vi "BioFeedback7(DAQ+8-channel)SubVIToUI.vi"(0 "UI Data Input File":path=path "C:/Users/Tinggroup/Desktop/VRMuscleActivationVisualizer/StationaryVisualFeedbackVR/assets/BiofeedbackData.txt", 7 "Frames Per Second":dbl=30.0, 9 "Start Trial":bool, 11 "End Trial":bool, 12 "Data Directory":path, 13 "File Name":string, 14 "Extension":string="_EMG.txt") -> ()   [LabVIEW 2016]
uses:
  <vilib>/Utility/error.llb/DialogType.ctl
  <vilib>/Analysis/5stat.llb/RMS (DBL).vi
  <vilib>/Waveform/WDTFileIO.llb/Export Waveform To Spreadsheet File.vi
  <vilib>/Waveform/WDTOps.llb/WDT Append Waveforms DBL.vi
  <vilib>/Analysis/NI_AALPro.lvlib
  <resource>/objmgr/daqmx.rc
panel:
  in  "EMG Input Device\nProduct Type":string
  out "Moving Avg 1AND2":dbl(slide) scale=0.0..0.01
  out "Moving Avg 3AND4":dbl(slide) scale=0.5..0.7
  out "RMS 3AND4":dbl(graph)
  out "RMS 1AND2":dbl(graph)
  out "RMS 8":dbl(graph)
  out "RMS 7":dbl(graph)
  out "RMS 6":dbl(graph)
  out "RMS 5":dbl(graph)
  out "RMS 4":dbl(graph)
  out "RMS 3":dbl(graph)
  out "RMS 2":dbl(graph)
  out "RMS 1":dbl(graph)
  out "Aggregate8":waveform(dbl)[](array[waveform])
  out "Aggregate7":waveform(dbl)[](array[waveform])
  out "Aggregate6":waveform(dbl)[](array[waveform])
  out "Aggregate5":waveform(dbl)[](array[waveform])
  out "Aggregate4":waveform(dbl)[](array[waveform])
  out "Aggregate3":waveform(dbl)[](array[waveform])
  out "Aggregate2":waveform(dbl)[](array[waveform])
  out "Aggregate1":waveform(dbl)[](array[waveform])
  out "Wfm8":waveform(dbl)
  out "Wfm7":waveform(dbl)
  out "Wfm6":waveform(dbl)
  out "Wfm5":waveform(dbl)
  out "Wfm4":waveform(dbl)
  out "Wfm3":waveform(dbl)
  out "Wfm2":waveform(dbl)
  out "Wfm1":waveform(dbl)
  out "Trial Data":waveform(dbl)(graph)
  in  "UI Percent Path":path=path "C:/Users/Tinggroup/Desktop/VRMuscleActivationVisualizer/StationaryVisualFeedbackVR/assets/BiofeedbackTargetPercentage.txt"
  in  "Target Percentage":dbl
  out "Trial In Progress":bool
  in  "Trial Number":dbl
  in  "MARK":bool
  out "Moving Avg RMS Graph":dbl(graph)
  out "Moving Avg RMS":dbl(slide) scale=0.0..2.0
  in  "Lower Cut-Off":dbl=20.0
  in  "Upper Cut-Off":dbl=300.0
  out "raw data":dynamicdata(graph)
  out "Bufffer Index":dbl
  out "Frames in Buffer":dbl
  out "Samples per frame":dbl
  out "Reset Data Acquisition\nAnd UI Updating":bool=TRUE
  in  "Moving Average Length (s)":dbl=0.5
  in  "Sample rate (Hz)":dbl=2000.0
  in  "End Program":bool
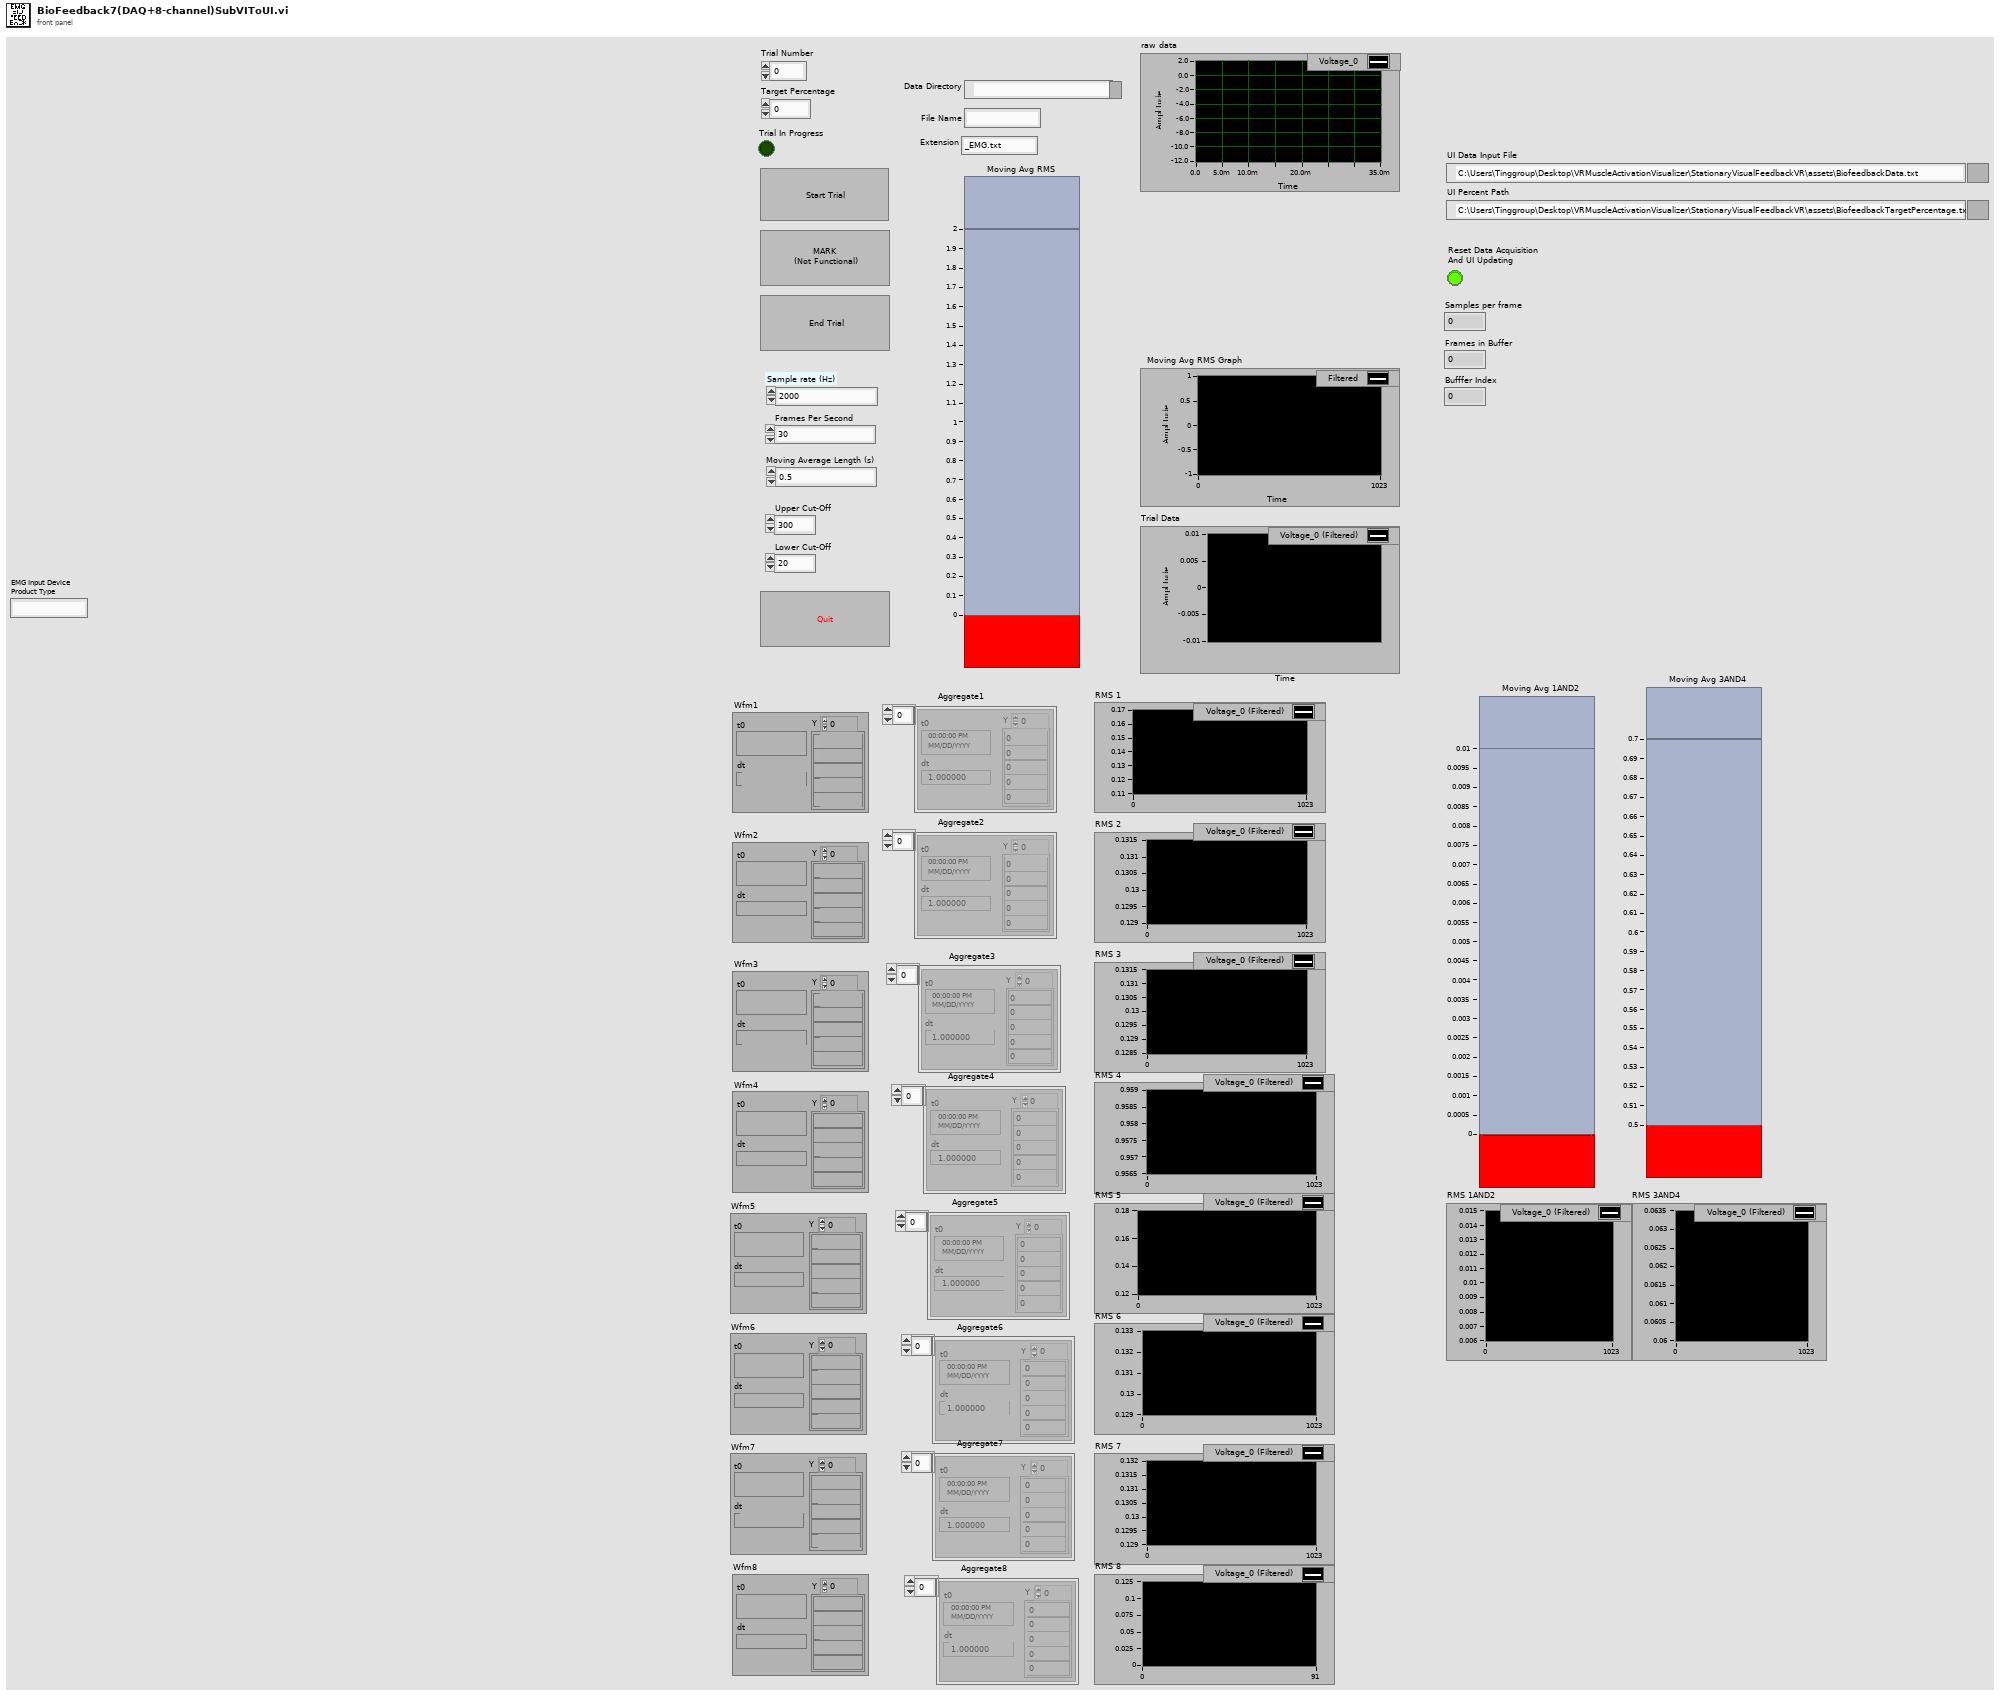
[diagram p1: front panel]
types:
  T1 = typedef "DialogType.ctl" = u16
  T2 = typedef "WaveformArrayControl.ctl" = waveform(dbl)[]
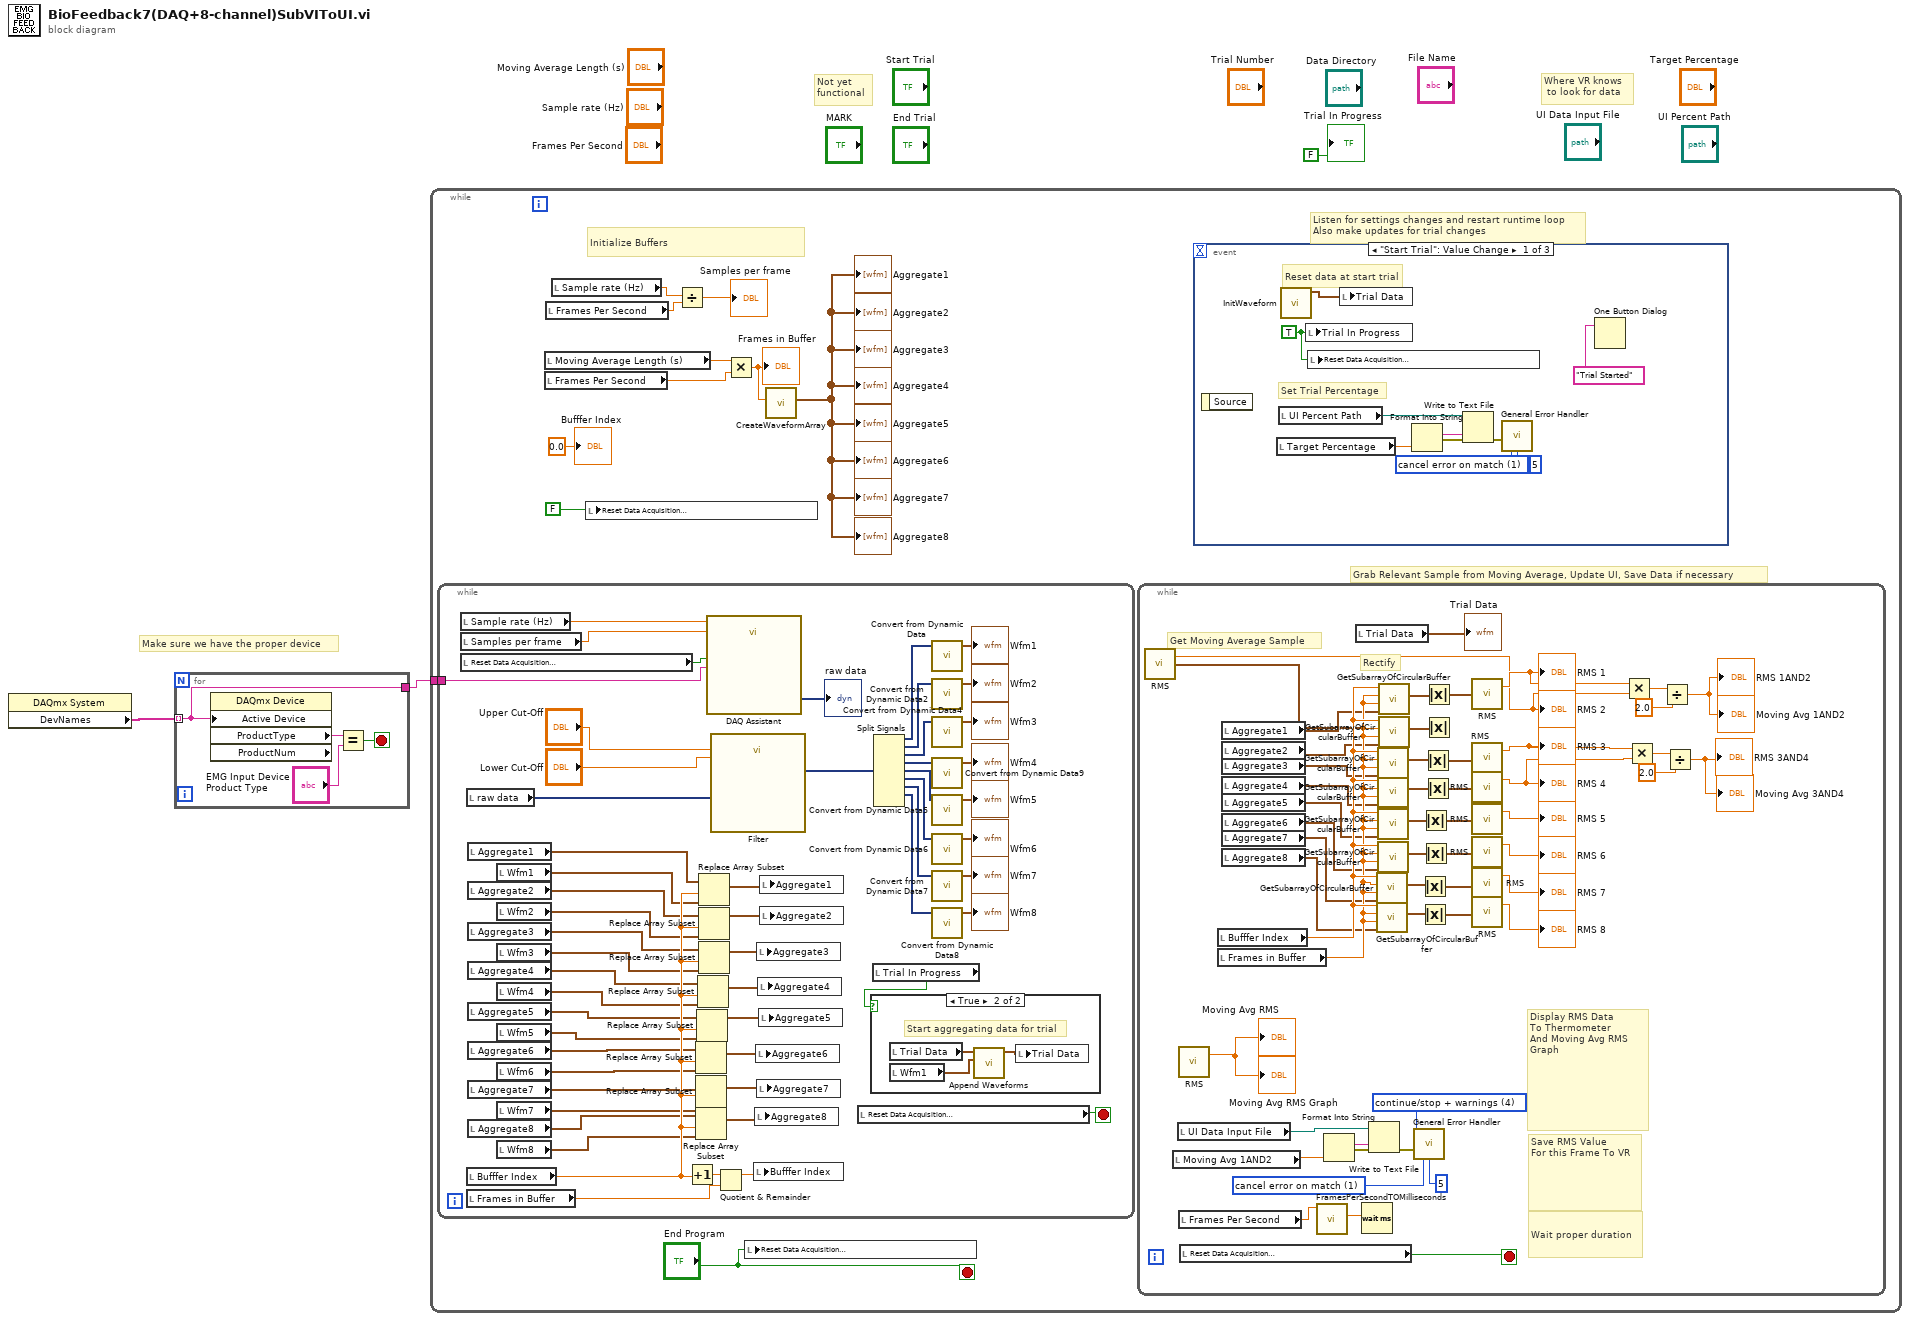
[diagram p0: block diagram]
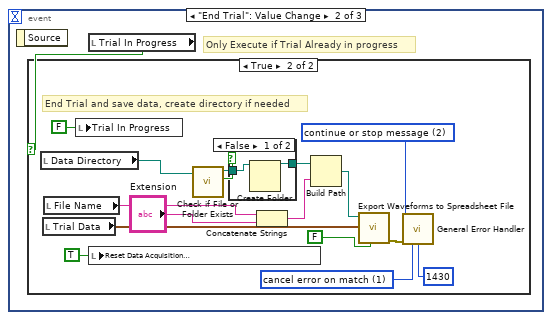
[diagram p2: hidden frame]
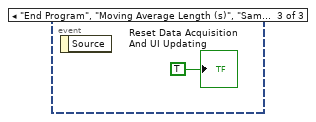
[diagram p5: hidden frame]
diagram:
  # "Make sure we have the proper device"
  # "Not yet \nfunctional"
  # "Where VR knows\n to look for data"
  n1 = property class="DAQmx System"() -> ("DevNames"=w2:tag[])  [unwired: 2 in, 2 out]
  n2 = for {
    tunnel: w2 -> [w4] mode=indexing
    tunnel: [w4] -> w1
    stop <- w5 stop-if-true
    n3 = property class="DAQmx Device" props=["Active Device", "ProductType", "ProductNum"]("Active Device"=w4) -> ("ProductType"=w7:string)  [unwired: 2 in, 3 out]
    n4 = Equal?(x=w7, y="EMG Input Device\nProduct Type") -> (x = y?=w5:bool)
  }
  n5 = while {
    tunnel: w1 -> [w8]
    stop <- "End Program" stop-if-true
    # "Grab Relevant Sample from Moving Average, Update UI, Save Data if necessary"
    # "Initialize Buffers"
    # "Listen for settings changes and restart runtime loop\nAlso make updates for trial changes"
    n6 = while {
      tunnel: w8 -> [w103]
      stop <- w149 stop-if-true
      n7 = local read "Sample rate (Hz)"() -> (w157:dbl)
      n8 = local read "Samples per frame"() -> (w156:dbl)
      n9 = local read "Reset Data Acquisition\nAnd UI Updating"() -> (w148:bool)
      n10 = local read "raw data"() -> (w154:dynamicdata)
      n11 = local read "Bufffer Index"() -> (w129:dbl)
      n12 = local read "Frames in Buffer"() -> (w151:dbl)
      n13 = local read "Aggregate1"() -> (w128:waveform(dbl)[])
      n14 = local read "Aggregate2"() -> (w126:waveform(dbl)[])
      n15 = local read "Aggregate3"() -> (w124:waveform(dbl)[])
      n16 = local read "Aggregate4"() -> (w122:waveform(dbl)[])
      n17 = local read "Aggregate5"() -> (w120:waveform(dbl)[])
      n18 = local read "Aggregate6"() -> (w118:waveform(dbl)[])
      n19 = local read "Aggregate7"() -> (w116:waveform(dbl)[])
      n20 = local read "Aggregate8"() -> (w114:waveform(dbl)[])
      n21 = local read "Wfm1"() -> (w127:waveform(dbl))
      n22 = local read "Wfm2"() -> (w125:waveform(dbl))
      n23 = local read "Wfm3"() -> (w123:waveform(dbl))
      n24 = local read "Wfm4"() -> (w121:waveform(dbl))
      n25 = local read "Wfm5"() -> (w119:waveform(dbl))
      n26 = local read "Wfm6"() -> (w117:waveform(dbl))
      n27 = local read "Wfm7"() -> (w115:waveform(dbl))
      n28 = local read "Wfm8"() -> (w113:waveform(dbl))
      n29 = Increment(x=w129) -> (x+1=w150:dbl)
      n30 = Replace Array Subset(array=w118, new element=w117, index=w129) -> (w107:waveform(dbl)[])
      n31 = Replace Array Subset(array=w116, new element=w115, index=w129) -> (w106:waveform(dbl)[])
      n32 = Replace Array Subset(array=w114, new element=w113, index=w129) -> (w105:waveform(dbl)[])
      n33 = Replace Array Subset(array=w120, new element=w119, index=w129) -> (w108:waveform(dbl)[])
      n34 = Replace Array Subset(array=w122, new element=w121, index=w129) -> (w109:waveform(dbl)[])
      n35 = Replace Array Subset(array=w128, new element=w127, index=w129) -> (w112:waveform(dbl)[])
      n36 = Replace Array Subset(array=w126, new element=w125, index=w129) -> (w111:waveform(dbl)[])
      n37 = Replace Array Subset(array=w124, new element=w123, index=w129) -> (w110:waveform(dbl)[])
      n38 = call "DAQ Assistant"("rate"=w157, "number of samples"=w156, "stop (T)"=w148, "device name"=w103) -> ("data"=→"raw data":dynamicdata)  [unwired: 13 in, 2 out]
      n39 = call "Filter"("Lower Cut-Off"="Lower Cut-Off", "Upper Cut-Off"="Upper Cut-Off", "Signal"=w154) -> ("Filtered Signal"=w146:dynamicdata)  [unwired: 7 in, 1 out]
      n40 = Quotient & Remainder(x=w150, y=w151) -> (x-y*floor(x/y)=w152:dbl)  [unwired: 1 out]
      n41 = local write "Bufffer Index"(w152) -> ()
      n42 = local write "Aggregate8"(w105) -> ()
      n43 = local write "Aggregate6"(w107) -> ()
      n44 = local write "Aggregate3"(w110) -> ()
      n45 = local write "Aggregate7"(w106) -> ()
      n46 = local write "Aggregate4"(w109) -> ()
      n47 = local write "Aggregate5"(w108) -> ()
      n48 = local write "Aggregate1"(w112) -> ()
      n49 = local write "Aggregate2"(w111) -> ()
      n50 = local read "Reset Data Acquisition\nAnd UI Updating"() -> (w149:bool)
      n51 = local read "Trial In Progress"() -> (w104:bool)
      n52 = case shown="True" w104 {
        frame False {
        }
        frame True {
          # "Start aggregating data for trial"
          n53 = local read "Trial Data"() -> (w160:waveform(dbl))
          n54 = local read "Wfm1"() -> (w159:waveform(dbl))
          n55 = call-poly <vilib>:"Append Waveforms.vi"("waveform B"=w159, "waveform A"=w160) -> ("waveform out"=w158:waveform(dbl))  [unwired: 8 in, 1 out]
          n56 = local write "Trial Data"(w158) -> ()
        }
      }
      n57 = Split Signals(w146) -> (w145:dynamicdata, w144:dynamicdata, w143:dynamicdata, w142:dynamicdata, w141:dynamicdata, w140:dynamicdata, w139:dynamicdata, w138:dynamicdata)  [unwired: 9 in, 1 out]
      n58 = call "Convert from Dynamic Data"("Dynamic Data Type"=w145) -> ("Waveform"=→"Wfm1":waveform(dbl))  [unwired: 3 in]
      n59 = call "Convert from Dynamic Data2"("Dynamic Data Type"=w144) -> ("Waveform"=→"Wfm2":waveform(dbl))  [unwired: 3 in]
      n60 = call "Convert from Dynamic Data4"("Dynamic Data Type"=w143) -> ("Waveform"=→"Wfm3":waveform(dbl))  [unwired: 3 in]
      n61 = call "Convert from Dynamic Data9"("Dynamic Data Type"=w142) -> ("Waveform"=→"Wfm4":waveform(dbl))  [unwired: 3 in]
      n62 = call "Convert from Dynamic Data5"("Dynamic Data Type"=w141) -> ("Waveform"=→"Wfm5":waveform(dbl))  [unwired: 3 in]
      n63 = call "Convert from Dynamic Data6"("Dynamic Data Type"=w140) -> ("Waveform"=→"Wfm6":waveform(dbl))  [unwired: 3 in]
      n64 = call "Convert from Dynamic Data7"("Dynamic Data Type"=w139) -> ("Waveform"=→"Wfm7":waveform(dbl))  [unwired: 3 in]
      n65 = call "Convert from Dynamic Data8"("Dynamic Data Type"=w138) -> ("Waveform"=→"Wfm8":waveform(dbl))  [unwired: 3 in]
    }
    n66 = local read "Moving Average Length (s)"() -> (w15:dbl)
    n67 = local read "Frames Per Second"() -> (w14:dbl)
    n68 = local read "Frames Per Second"() -> (w17:dbl)
    n69 = local read "Sample rate (Hz)"() -> (w18:dbl)
    n70 = local write "Reset Data Acquisition\nAnd UI Updating"(FALSE) -> ()
    n71 = Divide(x=w18, y=w17) -> (x/y=→"Samples per frame":dbl)
    n72 = Multiply(x=w15, y=w14) -> (x*y=w11:dbl)
    "Frames in Buffer" <- w11
    n73 = local write "Reset Data Acquisition\nAnd UI Updating"("End Program") -> ()
    n74 = call "CreateWaveformArray.vi"("bufferSize"=w11) -> ("initialized array"=→"Aggregate1" →"Aggregate2" →"Aggregate3" →"Aggregate4" →"Aggregate5" →"Aggregate6" →"Aggregate7" →"Aggregate8":waveform(dbl)[])  [unwired: 5 in, 1 out]
    n75 = while {
      stop <- w102 stop-if-true
      w90 = T1 4 items=["no dialog", "OK message", "continue or stop message", "OK message + warnings", "continue/stop + warnings"] ("type of dialog (OK msg:1)")
      w98 = 1 items=["no exception", "cancel error on match", "set error on match"] ("[exception action] (none:0)")
      # "Wait proper duration"
      # "Save RMS Value\nFor this Frame To VR"
      # "Display RMS Data\nTo Thermometer\nAnd Moving Avg RMS\nGraph"
      # "Get Moving Average Sample"
      # "Rectify"
      n76 = local read "Moving Avg 1AND2"() -> (w92:dbl)
      n77 = local read "UI Data Input File"() -> (w94:path)
      n78 = call-poly <vilib>:"RMS.vi"() -> ("rms value"=→"Moving Avg RMS" →"Moving Avg RMS Graph":dbl)  [unwired: 1 in, 1 out]
      n79 = local read "Frames Per Second"() -> (w100:dbl)
      n80 = local read "Reset Data Acquisition\nAnd UI Updating"() -> (w102:bool)
      n81 = local read "Bufffer Index"() -> (w89:dbl)
      n82 = local read "Frames in Buffer"() -> (w88:dbl)
      n83 = local read "Aggregate1"() -> (w87:waveform(dbl)[])
      n84 = local read "Aggregate2"() -> (w83:waveform(dbl)[])
      n85 = local read "Aggregate3"() -> (w86:waveform(dbl)[])
      n86 = local read "Aggregate4"() -> (w82:waveform(dbl)[])
      n87 = local read "Aggregate5"() -> (w85:waveform(dbl)[])
      n88 = local read "Aggregate6"() -> (w84:waveform(dbl)[])
      n89 = local read "Aggregate7"() -> (w81:waveform(dbl)[])
      n90 = local read "Aggregate8"() -> (w80:waveform(dbl)[])
      n91 = call "FramesPerSecondTOMilliseconds.vi"("Thermometer\nFps"=w100) -> ("x*y"=w99:dbl)  [unwired: 10 in]
      n92 = Format Into String(w92) -> (resulting string=w93:string, error out=w95:errorcluster)  [unwired: 3 in]
      n93 = local read "Trial Data"() -> (→"Trial Data":waveform(dbl))
      n94 = Wait (ms)(milliseconds to wait=w99) -> ()  [unwired: 1 out]
      n95 = Write to Text File(file (use dialog)=w94, text=w93, error in=w95) -> (error out=w96:errorcluster)  [unwired: 1 in, 2 out]
      n96 = call "GetSubarrayOfCircularBuffer.vi"("initialized array"=w81, "buffer size"=w88, "subset size"=w88, "start index"=w89) -> ("initialized array 2"=w73:T2)  [unwired: 7 in]
      n97 = call "GetSubarrayOfCircularBuffer.vi"("initialized array"=w80, "buffer size"=w88, "subset size"=w88, "start index"=w89) -> ("initialized array 2"=w72:T2)  [unwired: 7 in]
      n98 = call "GetSubarrayOfCircularBuffer.vi"("initialized array"=w86, "buffer size"=w88, "subset size"=w88, "start index"=w89) -> ("initialized array 2"=w77:T2)  [unwired: 7 in]
      n99 = call "GetSubarrayOfCircularBuffer.vi"("initialized array"=w82, "buffer size"=w88, "subset size"=w88, "start index"=w89) -> ("initialized array 2"=w76:T2)  [unwired: 7 in]
      n100 = call "GetSubarrayOfCircularBuffer.vi"("initialized array"=w85, "buffer size"=w88, "subset size"=w88, "start index"=w89) -> ("initialized array 2"=w75:T2)  [unwired: 7 in]
      n101 = call "GetSubarrayOfCircularBuffer.vi"("initialized array"=w84, "buffer size"=w88, "subset size"=w88, "start index"=w89) -> ("initialized array 2"=w74:T2)  [unwired: 7 in]
      n102 = call "GetSubarrayOfCircularBuffer.vi"("initialized array"=w87, "buffer size"=w88, "subset size"=w88, "start index"=w89) -> ("initialized array 2"=w79:T2)  [unwired: 7 in]
      n103 = call "GetSubarrayOfCircularBuffer.vi"("initialized array"=w83, "buffer size"=w88, "subset size"=w88, "start index"=w89) -> ("initialized array 2"=w78:T2)  [unwired: 7 in]
      n104 = call <vilib>:"General Error Handler.vi"("type of dialog (OK msg:1)"=w90, "error in (no error)"=w96, "[exception action] (none:0)"=w98, "[exception code]"=5) -> ()  [unwired: 7 in, 5 out]
      n105 = Absolute Value(x=w73) -> (abs(x)=w65:T2)
      n106 = Absolute Value(x=w72) -> (abs(x)=w64:T2)
      n107 = Absolute Value(x=w75) -> (abs(x)=w67:T2)
      n108 = Absolute Value(x=w74) -> (abs(x)=w66:T2)
      n109 = Absolute Value(x=w77) -> (abs(x)=w69:T2)
      n110 = Absolute Value(x=w76) -> (abs(x)=w68:T2)
      n111 = Absolute Value(x=w79) -> (abs(x)=w71:T2)
      n112 = Absolute Value(x=w78) -> (abs(x)=w70:T2)
      n113 = call-poly <vilib>:"RMS.vi"("X"=w70) -> ("rms value"=w58:dbl)  [unwired: 1 out]
      "RMS 2" <- w58
      n114 = call-poly <vilib>:"RMS.vi"("X"=w71) -> ("rms value"=w59:dbl)  [unwired: 1 out]
      "RMS 1" <- w59
      n115 = call-poly <vilib>:"RMS.vi"("X"=w69) -> ("rms value"=w53:dbl)  [unwired: 1 out]
      "RMS 3" <- w53
      n116 = call-poly <vilib>:"RMS.vi"("X"=w68) -> ("rms value"=w52:dbl)  [unwired: 1 out]
      "RMS 4" <- w52
      n117 = call-poly <vilib>:"RMS.vi"("X"=w67) -> ("rms value"=→"RMS 5":dbl)  [unwired: 1 out]
      n118 = call-poly <vilib>:"RMS.vi"("X"=w66) -> ("rms value"=→"RMS 6":dbl)  [unwired: 1 out]
      n119 = call-poly <vilib>:"RMS.vi"("X"=w65) -> ("rms value"=→"RMS 7":dbl)  [unwired: 1 out]
      n120 = call-poly <vilib>:"RMS.vi"("X"=w64) -> ("rms value"=→"RMS 8":dbl)  [unwired: 1 out]
      n121 = Multiply(x=w59, y=w58) -> (x*y=w57:dbl)
      n122 = Multiply(x=w53, y=w52) -> (x*y=w55:dbl)
      n123 = Divide(x=w57, y=2.0) -> (x/y=→"RMS 1AND2" →"Moving Avg 1AND2":dbl)
      n124 = Divide(x=w55, y=2.0) -> (x/y=→"RMS 3AND4" →"Moving Avg 3AND4":dbl)
    }
    n125 = event shown="[0] \"Start Trial\": Value Change" {
      selector: _ -> [_ _ _]
      dyn-events: _ -> [_ _ _]
      timeout: _ -> [_ _ _]
      event "Start Trial": Value Change {
        w26 = 1 items=["no exception", "cancel error on match", "set error on match"] ("[exception action] (none:0)")
        w27 = TRUE ("Trial In Progress")
        # "Set Trial Percentage"
        # "Reset data at start trial"
        n126 = event-data() -> ()  [unwired: 1 in, 1 out]
        n127 = local read "Target Percentage"() -> (w20:dbl)
        n128 = local read "UI Percent Path"() -> (w21:path)
        n129 = call "InitWaveform.vi"() -> ("output waveform"=w28:waveform(dbl))  [unwired: 11 in]
        n130 = local write "Trial In Progress"(w27) -> ()
        n131 = local write "Reset Data Acquisition\nAnd UI Updating"(w27) -> ()
        n132 = local write "Trial Data"(w28) -> ()
        n133 = Format Into String(w20) -> (resulting string=w22:string, error out=w23:errorcluster)  [unwired: 3 in]
        n134 = Write to Text File(file (use dialog)=w21, text=w22, error in=w23) -> (error out=w24:errorcluster)  [unwired: 1 in, 2 out]
        n135 = call <vilib>:"General Error Handler.vi"("error in (no error)"=w24, "[exception action] (none:0)"=w26, "[exception code]"=5) -> ()  [unwired: 8 in, 5 out]
        n136 = One Button Dialog(message="Trial Started") -> ()  [unwired: 1 in, 1 out]
      }
      event "End Trial": Value Change {
        # "Only Execute if Trial Already in progress"
        n137 = event-data() -> ()  [unwired: 1 in, 1 out]
        n138 = local read "Trial In Progress"() -> (w29:bool)
        n139 = case shown="True" w29 {
          frame False {
          }
          frame True {
            w38 = T1 2 items=["no dialog", "OK message", "continue or stop message", "OK message + warnings", "continue/stop + warnings"] ("type of dialog (OK msg:1)")
            w39 = 1 items=["no exception", "cancel error on match", "set error on match"] ("[exception action] (none:0)")
            # "End Trial and save data, create directory if needed"
            n140 = local read "Data Directory"() -> (w41:path)
            n141 = local read "Trial Data"() -> (w33:waveform(dbl))
            n142 = local read "File Name"() -> (w36:string)
            n143 = local write "Trial In Progress"(FALSE ("Trial In Progress")) -> ()
            n144 = local write "Reset Data Acquisition\nAnd UI Updating"(TRUE ("Reset Data Acquisition\nAnd UI Updating")) -> ()
            n145 = call <vilib>:"Check if File or Folder Exists.vi"("path"=w41) -> ("file or folder exists?"=w43:bool, "dup path"=w42:path)  [unwired: 8 in, 1 out]
            n146 = case shown="False" w43 {
              tunnel: [w46 w48] -> w34
              tunnel: w42 -> [w47 w48]
              frame False {
                n147 = Create Folder(path (use dialog)=w47) -> (created path=w46:path)  [unwired: 2 in, 2 out]
              }
              frame True {
              }
            }
            n148 = Concatenate Strings(w36, "Extension") -> (w35:string)
            n149 = Build Path(base path=w34, name or relative path=w35) -> (appended path=w32:path)
            n150 = call-poly <vilib>:"Export Waveforms to Spreadsheet File.vi"("append to file? (new file:F)"=FALSE, "waveform"=w33, "file path (dialog if empty)"=w32) -> ("error out"=w31:errorcluster)  [unwired: 7 in, 1 out]
            n151 = call <vilib>:"General Error Handler.vi"("type of dialog (OK msg:1)"=w38, "error in (no error)"=w31, "[exception action] (none:0)"=w39, "[exception code]"=1430) -> ()  [unwired: 7 in, 5 out]
          }
        }
      }
      event "End Program", "Moving Average Length (s)", "Sample rate (Hz)", "Frames Per Second": Value Change {
        n152 = event-data() -> ()  [unwired: 1 in, 1 out]
        "Reset Data Acquisition\nAnd UI Updating" <- TRUE
      }
    }
    "Bufffer Index" <- 0.0 ("Bufffer Index")
  }
  "Trial In Progress" <- FALSE ("Trial In Progress")
